vi "AVI.vi"() -> ()   [LabVIEW 2014]
doc: "This example shows how to open, read, and display an AVI file in NI Vision. The VI reads the frames per second property and plays the images back at the rate specified by the AVI file."
uses:
  <vilib>/Utility/miscctls.llb/LVRectTypeDef.ctl
  <resource>/objmgr/IMAQImage.rc
panel:
  out "Front Panel Window:Window Bounds":T1
  out "Image Area:Size:All Elements":cluster{"Width":u32, "Height":u32}
  out "Image Size":cluster{"x":i32, "y":i32}
  out "Progress Bar":i32(slide) max=115 scale=1.0..115.0
  in  "Stop":bool
  out "Image":T2(plugin-control)
  # "Overview: Demonstrate the use of the AVI functions to read an AVI movie file.\nRequirements: Vision Development Software.\nInstructions: Run the VI."
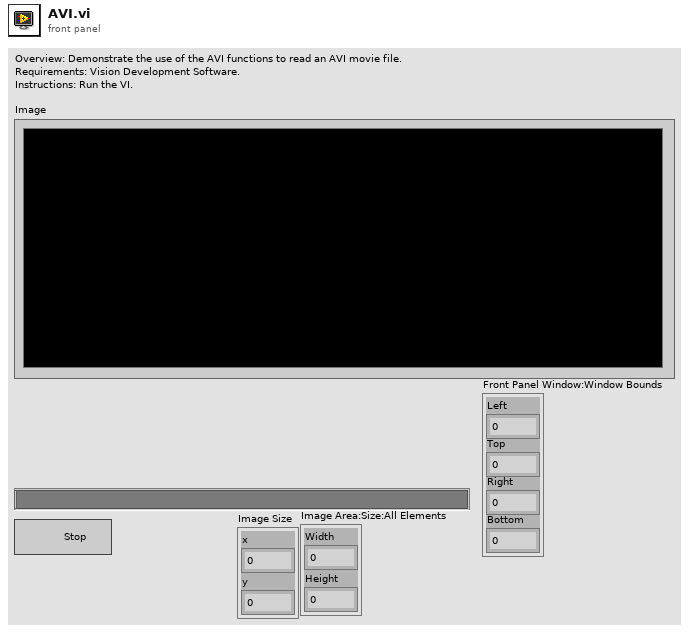
[diagram p1: front panel]
types:
  T1 = typedef "LVRectTypeDef.ctl" = cluster{"Left":i16, "Top":i16, "Right":i16, "Bottom":i16}
  T2 = typedef "IMAQ Image.ctl" = refnum<image>
  T3 = typedef "IMAQ AVI2 Refnum.ctl" = refnum<k20>
  T4 = typedef "Image Type" = u32
  T5 = cluster{"Width":u32, "Height":u32, "Frames Per Second":u32, "Codec":string, "Has Data":bool}
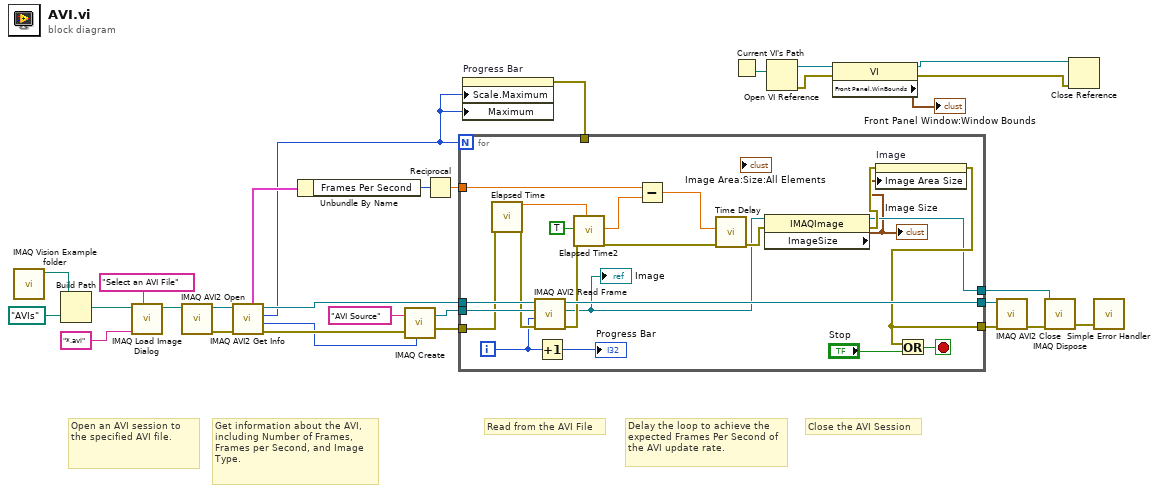
[diagram p0: block diagram]
diagram:
  # "Close the AVI Session"
  # "Read from the AVI File"
  # "Get information about the AVI, including Number of Frames, Frames per Second, and Image Type."
  # "Open an AVI session to the specified AVI file."
  # "Delay the loop to achieve the expected Frames Per Second of the AVI update rate."
  n1 = call "IMAQ Vision Example folder.vi"() -> ("Example Image Path"=w14:path)  [unwired: 11 in]
  n2 = Build Path(base path=w14, name or relative path=path "AVIs") -> (appended path=w11:path)
  n3 = call "IMAQ Load Image Dialog"("Prompt"="Select an AVI File" ("prompt"), "Pattern"="*.avi", "Start Path"=w11) -> ("Path"=w10:path)  [unwired: 6 in, 2 out]
  n4 = call "IMAQ AVI2 Open"("AVI File Path"=w10) -> ("error out"=w27:errorcluster, "AVI Refnum"=w26:T3)  [unwired: 2 in, 7 out]
  n5 = call "IMAQ AVI2 Get Info"("error in (no error)"=w27, "AVI Refnum"=w26) -> ("error out"=w23:errorcluster, "Image Type"=w17:T4, "Number of Frames"=w8:u32, "AVI Refnum (duplicate)"=w20:T3, "Frame Data"=w28:T5)  [unwired: 5 out]
  n6 = Unbundle By Name(w28) -> ("Frames Per Second"=w16:u32)
  n7 = call "IMAQ Create"("Image Name"="AVI Source", "Image Type"=w17, "error in (no error)"=w23) -> ("New Image"=w21:T2, "error out"=w22:errorcluster)  [unwired: 1 in, 1 out]
  n8 = Reciprocal(x=w16) -> (1/x=w15:dbl)
  n9 = property on="Progress Bar" class="Slide (strict)"("Scale.Maximum"=w8, "Maximum"=w8) -> (error out=w7:errorcluster)  [unwired: 2 in, 1 out]
  n10 = for {
    N: w8 -> [_]
    tunnel: w21 -> [w51]
    tunnel: [w50] -> w24
    tunnel: [w33] -> w25
    tunnel: w22 -> [w49]
    tunnel: w20 -> [w52]
    tunnel: [w32] -> w18
    tunnel: w15 -> [w47]
    tunnel: w7 -> [_]
    i -> [w38]
    stop <- w39 stop-if-true
    n11 = call "Elapsed Time"("error in (no error)"=w49) -> ("Present (s)"=w45:dbl, "error out"=w48:errorcluster)  [unwired: 11 in, 6 out]
    n12 = call "IMAQ AVI2 Read Frame"("error in (no error)"=w48, "Frame Number"=w38, "Image"=w51, "AVI Refnum"=w52) -> ("error out"=w43:errorcluster, "Image Out"=w35:T2, "AVI Refnum (duplicate)"=w50:T3)  [unwired: 5 out]
    "Image" <- w35
    n13 = Increment(x=w38) -> (x+1=→"Progress Bar":i32)
    n14 = call "Elapsed Time2"("Reset"=TRUE, "error in (no error)"=w43, "Set Start Time (s)"=w45) -> ("Elapsed Time (s)"=w42:dbl, "error out"=w41:errorcluster)  [unwired: 9 in, 6 out]
    n15 = Subtract(x=w47, y=w42) -> (x-y=w46:dbl)
    n16 = call "Time Delay"("error in (no error)"=w41, "Delay Time (s)"=w46) -> ("error out"=w36:errorcluster)  [unwired: 9 in]
    n17 = property class="IMAQImage"(reference=w35, error in=w36) -> (reference out=w32:T2, error out=w34:errorcluster, "ImageSize"=w31:cluster{"x":i32, "y":i32})
    "Image Size" <- w31
    n18 = property on="Image" class="ImageControl"(error in=w34, "Image Area Size"=w31) -> (error out=w33:errorcluster)  [unwired: 1 in, 1 out]
    n19 = Or(x=w33, y="Stop") -> (x .or. y?=w39:bool)
  }
  n20 = Current VI's Path() -> (path=w6:path)
  n21 = Open VI Reference(vi path=w6) -> (vi reference=w5:refnum<vi>, error out=w4:errorcluster)  [unwired: 5 in]
  n22 = property class="VI"(reference=w5, error in=w4) -> (reference out=w3:refnum<vi>, error out=w2:errorcluster, "Front Panel.WinBounds"=→"Front Panel Window:Window Bounds":T1)
  n23 = call "IMAQ AVI2 Close"("error in (no error)"=w25, "AVI Refnum"=w24) -> ("error out"=w19:errorcluster)  [unwired: 9 out]
  n24 = call "IMAQ Dispose"("Image"=w18, "error in (no error)"=w19) -> ("error out"=w29:errorcluster)  [unwired: 1 in, 3 out]
  n25 = Close Reference(reference=w3, error in (no error)=w2) -> ()  [unwired: 1 out]
  n26 = call <vilib>:"Simple Error Handler.vi"("error in (no error)"=w29) -> ()  [unwired: 1 in, 8 out]
